vi "SCT Handle Main Loop Listener Event.vi"(4 "default types":T5, 5 "value":variant, 6 "feature pack info":T2, 7 "name":string, 8 "error in (no error)":errorcluster, 10 "state variable in":T7, 11 "Variable Dialog Controls in":T1) -> (0 "error out":errorcluster, 1 "Update Control States?":bool, 2 "state variables out":T7, 3 "Variable Dialog Controls out":T1)   [LabVIEW 2016]
uses:
  <resource>/dialog/variable/SCT Variable Dialog Controls.ctl
  <resource>/dialog/variable/SCT State Variables.ctl
  <resource>/dialog/variable/SCT Feature State.ctl
  <resource>/dialog/variable/SCT Variable Changes.ctl
  <vilib>/variable/Type Descriptor.ctl
  <resource>/dialog/variable/SCT Attribute Changes.ctl
  <resource>/dialog/variable/SCT Default Types.ctl
  <resource>/dialog/variable/SCT Feature Pack Info.ctl
  <resource>/dialog/variable/SCT Message User Event.ctl
  <resource>/dialog/variable/SCT Message.ctl
  <resource>/dialog/variable/SCT Attributes.ctl
  <resource>/dialog/variable/SCT Attributes Event.ctl
  <vilib>/variable/NI_Variable.lvlib
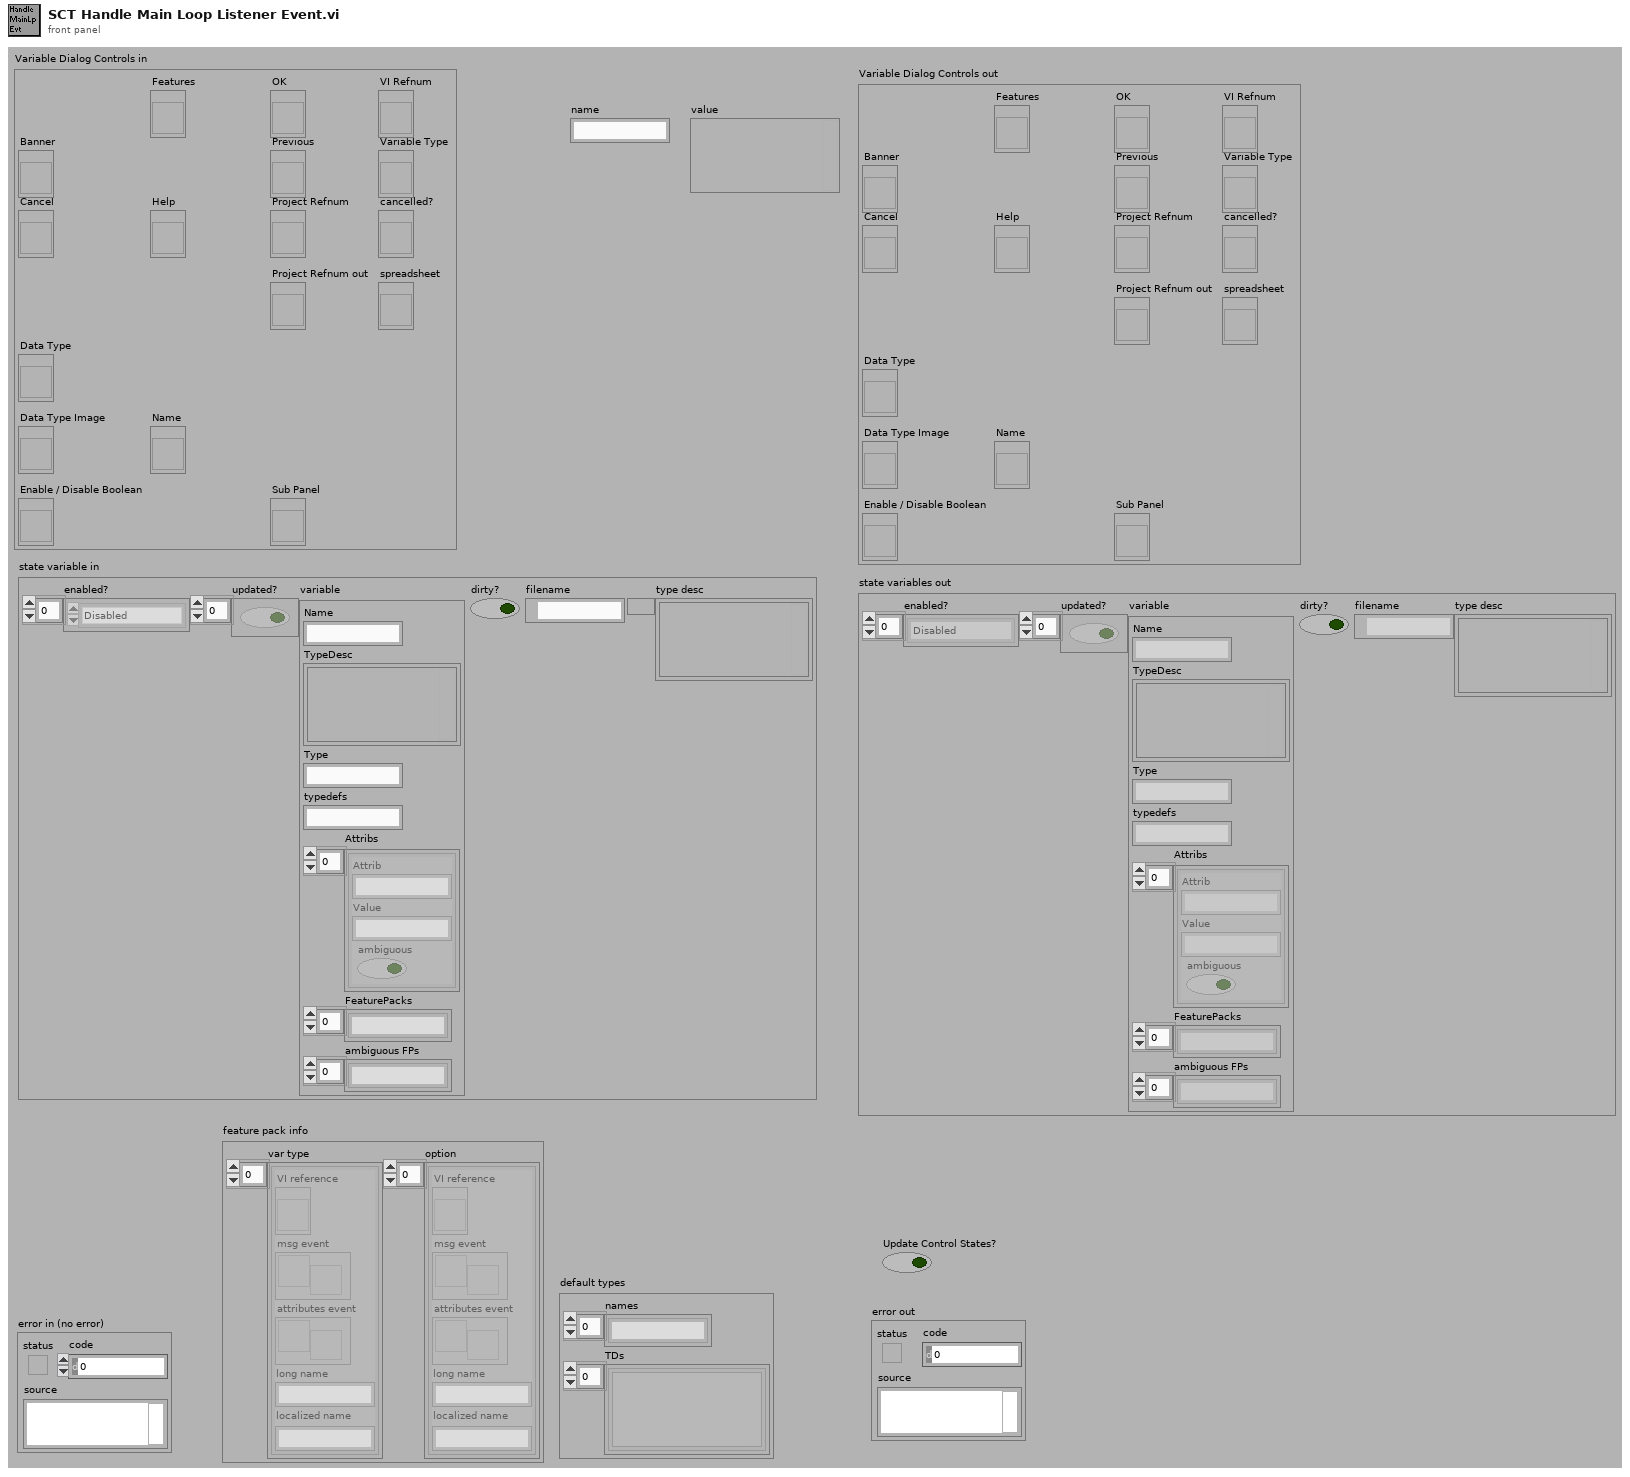
[diagram p1: front panel]
types:
  T1 = typedef "SCT Variable Dialog Controls.ctl" = cluster{"Banner":refnum<vi>, "Cancel":refnum<vi>, "Data Type":refnum<vi>, "Data Type Image":refnum<vi>, "Enable / Disable Boolean":refnum<vi>, "Features":refnum<vi>, "Help":refnum<vi>, "Name":refnum<vi>, "OK":refnum<vi>, "Previous":refnum<vi>, "Project Refnum":refnum<vi>, "Project Refnum out":refnum<vi>, "Sub Panel":refnum<vi>, "VI Refnum":refnum<vi>, "Variable Type":refnum<vi>, "cancelled?":refnum<vi>, "spreadsheet":refnum<vi>}
  T2 = typedef "SCT Feature Pack Info.ctl" = cluster{"var type":cluster{"VI reference":refnum<vi>, "msg event":T3, "attributes event":T4, "long name":string, "localized name":string}[], "option":cluster{"VI reference":refnum<vi>, "msg event":T3, "attributes event":T4, "long name":string, "localized name":string}[]}
  T3 = typedef "SCT Message User Event.ctl" = refnum<user-event>
  T4 = typedef "SCT Attributes Event.ctl" = refnum<user-event>
  T5 = typedef "SCT Default Types.ctl" = cluster{"names":string[], "TDs":T6[]}
  T6 = typedef "NI_Variable.lvlib/Type Descriptor.ctl" = cluster{"Variant":variant}
  T7 = typedef "SCT State Variables.ctl" = cluster{"enabled?":T8[], "updated?":bool[], "variable":T9, "dirty?":bool, "filename":path, "type desc":T6}
  T8 = typedef "SCT Feature State.ctl" = enum16{"Disabled", "Enabled", "Ambiguous", "Grayed", "MultiSelectConst"}
  T9 = typedef "SCT Variable Changes.ctl" = cluster{"Name":string, "TypeDesc":T6, "Type":string, "typedefs":string, "Attribs":T10, "FeaturePacks":string[], "ambiguous FPs":string[]}
  T10 = typedef "SCT Attribute Changes.ctl" = cluster{"Attrib":string, "Value":string, "ambiguous":bool}[]
  T11 = typedef "SCT Message.ctl" = cluster{"request type":enum16{"No Message", "New Data Type", "New Variable", "Request Values", "Shutdown", "Broadcast", "Show Help"}, "name":string, "type descriptor":T6, "scope":string, "attributes":T12, "broadcast value":variant}
  T12 = typedef "SCT Attributes.ctl" = cluster{"name":string, "value":string, "ambiguous?":bool}[]
  T13 = cluster{"VI reference":refnum<vi>, "msg event":T3, "attributes event":T4, "long name":string, "localized name":string}[]
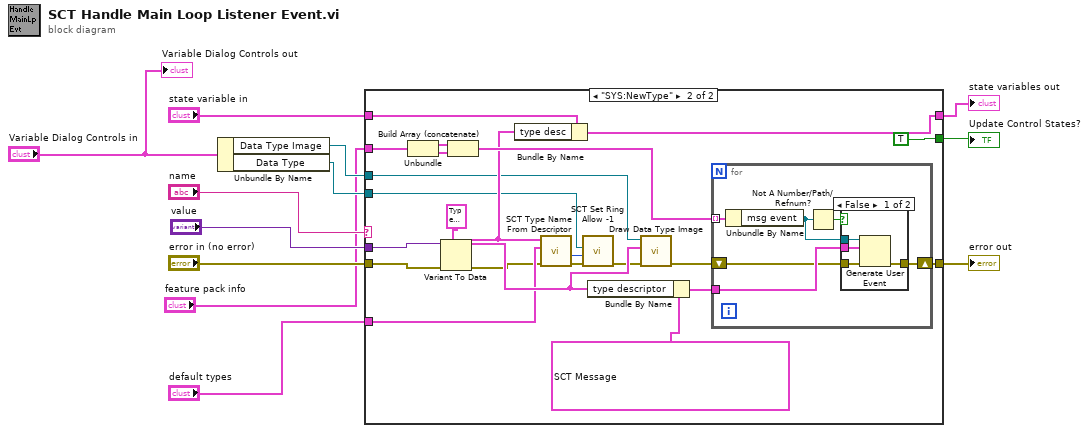
[diagram p0: block diagram]
diagram:
  n1 = Unbundle By Name("Variable Dialog Controls in") -> ("Data Type Image"=w11:refnum<vi>, "Data Type"=w12:refnum<vi>)
  n2 = case shown="\"SYS:NewType\"" "name" {
    tunnel: "feature pack info" -> [_ w36]
    tunnel: "value" -> [_ w31]
    tunnel: "default types" -> [_ w23]
    tunnel: [_ TRUE] -> w5
    tunnel: "state variable in" -> [w14 w26]
    tunnel: [w14 w25] -> w7
    tunnel: "error in (no error)" -> [w13 w18]
    tunnel: [w13 w19] -> w9
    tunnel: w11 -> [_ w16]
    tunnel: w12 -> [_ w15]
    frame "False", Default {
    }
    frame "SYS:NewType" {
      n3 = Unbundle(w36) -> ("var type"=w35:T13, "option"=w34:T13)
      n4 = Variant To Data(error in=w18, type=T6 {"Variant"=variant} ("type descriptor"), Variant=w31) -> (data=w24:T6, error out=w17:errorcluster)
      n5 = Build Array (concatenate)(w35, w34) -> (w33:T13)
      n6 = Bundle By Name(cluster=w26, "type desc"=w24) -> (w25:T7)
      n7 = call <resource>:"SCT Type Name From Descriptor.vi"("error in (no error)"=w17, "default types"=w23, "type descriptor"=w24) -> ("error out"=w21:errorcluster, "index to type"=w22:i32)  [unwired: 6 in, 1 out]
      n8 = call <resource>:"SCT Set Ring Allow -1.vi"("error in (no error)"=w21, "index"=w22, "ring"=w15) -> ("error out"=w20:errorcluster)  [unwired: 7 in, 1 out]
      n9 = Bundle By Name(cluster=T11 {"request type"=enum."New Data Type", "name"="", "type descriptor"={"Variant"=variant}, "scope"="", "attributes"=[], "broadcast value"=variant} ("event data"), "type descriptor"=w24) -> (w32:T11)
      n10 = call <vilib>:"Draw Data Type Image.vi"("error in (no error)"=w20, "type descriptor"=w24, "Data Type Image"=w16) -> ("error IO"=w28:errorcluster)  [unwired: 8 in]
      n11 = for {
        tunnel: w33 -> [w42] mode=indexing
        tunnel: w32 -> [w41]
        shift-right: [w37] -> w19
        shift-left: w28 -> [w38]
        n12 = Unbundle By Name(w42) -> ("msg event"=w40:T3)
        n13 = Not A Number/Path/Refnum?(number/path/refnum=w40) -> (NaN/Path/Refnum?=w39:bool)
        n14 = case shown="False" w39 {
          tunnel: w41 -> [w46 _]
          tunnel: w40 -> [w45 _]
          tunnel: w38 -> [w44 w47]
          tunnel: [w43 w47] -> w37
          frame False {
            n15 = Generate User Event(user event=w45, event data cluster=w46, error in=w44) -> (error out=w43:errorcluster)  [unwired: 1 in, 1 out]
          }
          frame True {
          }
        }
      }
    }
  }
  "error out" <- w9
  "state variables out" <- w7
  "Update Control States?" <- w5
  "Variable Dialog Controls out" <- "Variable Dialog Controls in"
